vi "Instrument - Manual Object.vi"() -> ()   [LabVIEW 2013, in "Instrument Workspace Objects.lvlib"]
doc: "Sample numeric display item."
uses:
  Instrument Workspace Objects.llb/Instrument Workspace Objects.lvlib
  NationalInstruments.VeriStand.SystemStorage
  Instrument Workspace Objects.llb/Instrument CD Host API.lvlib
panel:
  out "Device":string
  in  "NIVS.System Definition Root":refnum<k24>
  out "Error Report":errorcluster
  in  "Response?":bool
  out "Timed Out?":bool
  out "Response":string
  in  "Send":bool
  in  "Wait Value":dbl=100.0 format="%#_p"
  in  "Wait Type":enum16{"Byte Count", "Wait sec"}(ring)
  in  "Command":string
  in  "Item.Data":T1
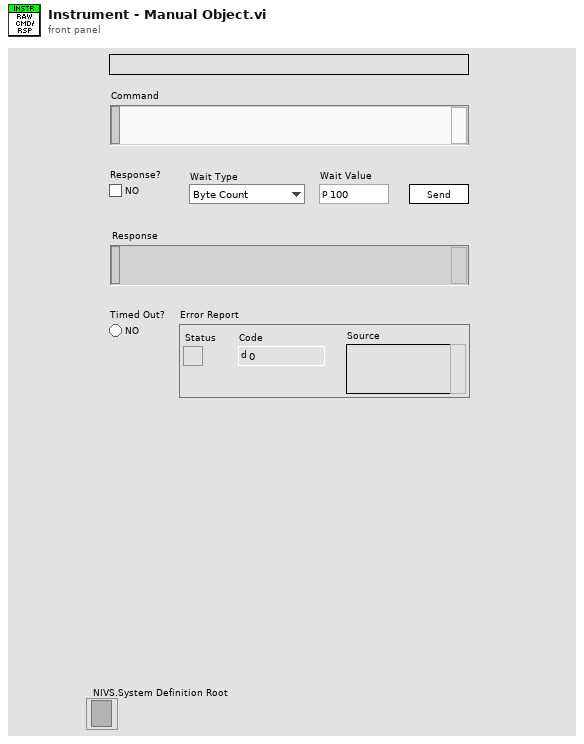
[diagram p1: front panel]
types:
  T1 = cluster{"Template VI":string, "Position X":i32, "Position Y":i32, "Custom":string, "Show Title Bar":bool, "ID":i32, "Always On Top":bool, "Allow Resize":bool, "Allow Minimize":bool, "Allow Close":bool, "Size to Screen":bool, "Screen.ID":i32, "State":enum16{"Normal", "New"}, "Title":string, "Window Bounds":cluster{"[0]":i16, "[1]":i16, "[2]":i16, "[3]":i16}, "Channel Ref":u64, "Unit":string, "Default Units?":bool, "Flash Limit?":bool, "Color 1":u32, "Color 2":u32, "Color 3":u32, "Color 4":u32, "Bck Color":u32, "Fore Color":u32, "Limit 1":dbl, "Limit 2":dbl, "Limit 3":dbl, "Limit 4":dbl, "Limit Mode 1":i32, "Limit Mode 2":i32, "Limit Mode 3":i32, "Limit Mode 4":i32, "Scale Precision":i32, "Scale Min":dbl, "Scale Max":dbl, "Format":i32, "Precision":i32, "Background Type":i32, "IDs":i32[], "Units":string[], "Labels":string[], "Scale Factor":dbl, "Scale Offset":dbl, "YScale Index":u32[], "XScale":cluster{"Format":u8, "Precision":u8, "Fit":u8, "Label":string, "Use Default Label":bool, "Label Visible":bool, "Min":dbl, "Max":dbl}, "YScales":cluster{"Format":u8, "Precision":u8, "Fit":u8, "Label":string, "Use Default Label":bool, "Label Visible":bool, "Min":dbl, "Max":dbl}[], "Plots":cluster{"Bar Style":u8, "Fill To":i16, "Fill/PtColor":u32, "Line Style":u8, "Line Width":u8, "Color":u32, "Interp":u8, "Point Style":u8}[], "Update Period":dbl, "History Length":dbl, "My.Ref":refnum<vi>, "Is Control?":bool, "Channel Paths":string[], "Custom Data":variant}
  T2 = cluster{"Operation":enum16{"SetCustomData", "DeleteItem"}, "Data":variant}
  T3 = cluster{"connection ID":refnum<k5>, "Meta data":string[]}
  T4 = cluster{"Command":string, "Response Expected?":bool, "Wait Type":enum16{"Byte Count", "Wait sec"}, "Wait Value":dbl}
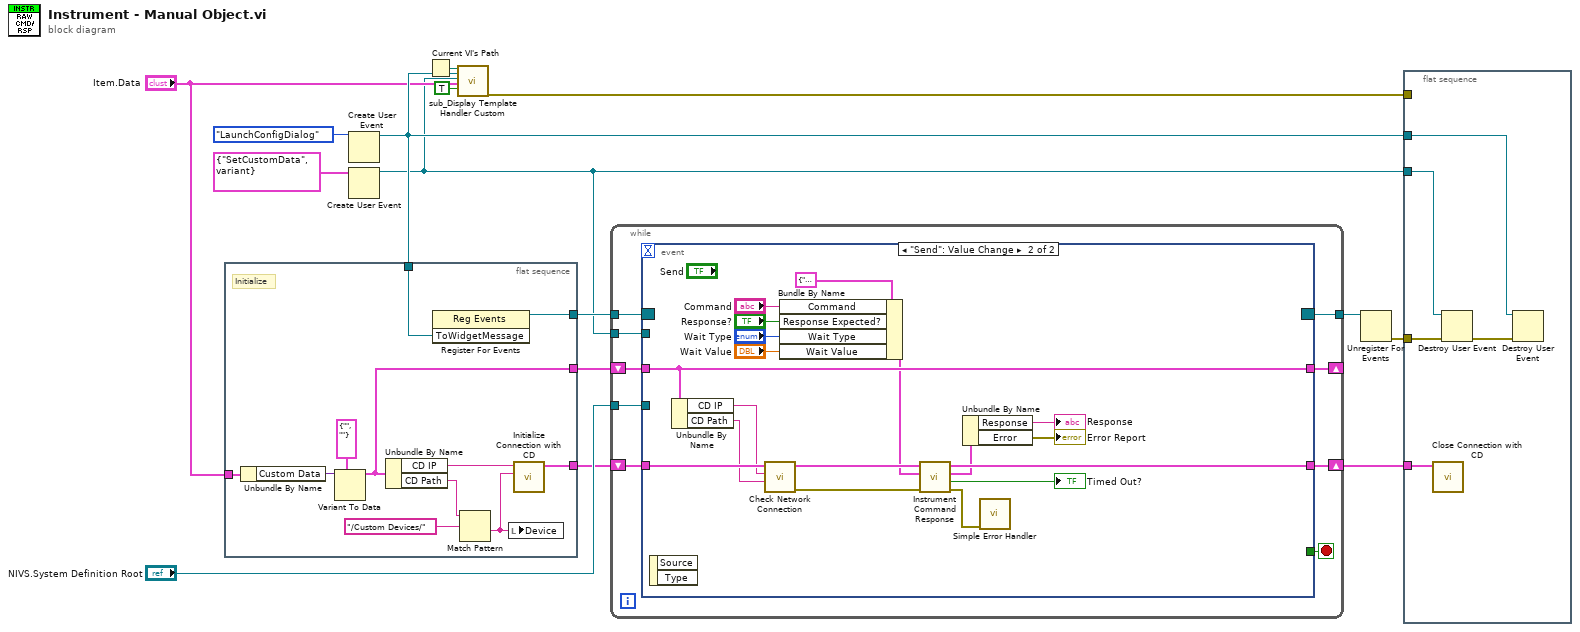
[diagram p0: block diagram]
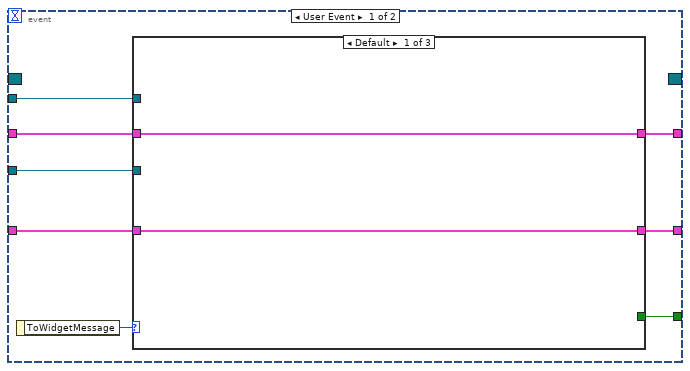
[diagram p2: hidden frame]
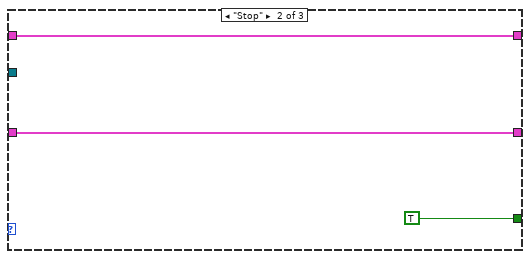
[diagram p3: hidden frame]
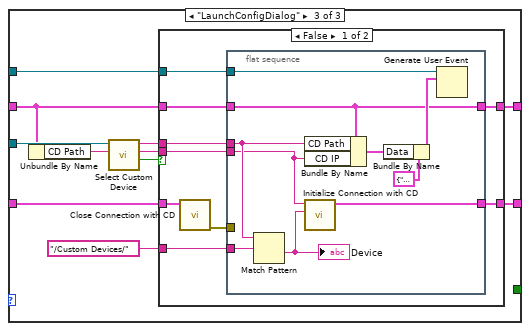
[diagram p4: hidden frame]
diagram:
  n1 = flat-sequence {
    tunnel: [w26] -> w13
    tunnel: w10 -> [w25]
    tunnel: "Item.Data" -> [w24]
    tunnel: [w17] -> w3
    tunnel: [w16] -> w2
    frame #0 {
      # "Initialize"
      n2 = Unbundle By Name(w24) -> ("Custom Data"=w23:variant)
      n3 = Variant To Data(type=cluster{"CD Path":string, "CD IP":string} {"CD Path"="", "CD IP"=""}, Variant=w23) -> (data=w17:cluster{"CD Path":string, "CD IP":string})  [unwired: 1 in, 1 out]
      n4 = Unbundle By Name(w17) -> ("CD IP"=w20:string, "CD Path"=w18:string)
      n5 = register-events(w25) -> (reference out=w26:refnum<event-registration>)  [unwired: 2 in, 1 out]
      n6 = Match Pattern(string=w18, regular expression="/Custom Devices/") -> (after substring=w19:string)  [unwired: 1 in, 3 out]
      n7 = local write "Device"(w19) -> ()
      n8 = call "Initialize Connection with CD.vi"("TCP Service"=w19, "IP Address"=w20) -> ("Connection Info Out"=w16:T3)  [unwired: 8 in, 1 out]
    }
  }
  n9 = Create User Event(user event datatype=enum16{"Stop", "LaunchConfigDialog"}."LaunchConfigDialog" ("ToWidgetMessage")) -> (user event=w10:refnum<user-event>)  [unwired: 1 in, 1 out]
  n10 = Create User Event(user event datatype=T2 {"Operation"=enum."SetCustomData", "Data"=variant} ("Data")) -> (user event=w6:refnum<user-event>)  [unwired: 1 in, 1 out]
  n11 = Current VI's Path() -> (path=w8:path)
  n12 = call "sub_Display Template Handler Custom.vi"("Parent.Path"=w8, "ToWidgetEvent"=w10, "ToWorkspace"=w6, "Item.Data"="Item.Data", "Resizable"=TRUE) -> ("error out"=w15:errorcluster)  [unwired: 14 in]
  n13 = while {
    tunnel: w13 -> [w35]
    tunnel: [w33] -> w12
    tunnel: w6 -> [w32]
    tunnel: "NIVS.System Definition Root" -> [w31]
    shift-right: [w27] -> _
    shift-left: w3 -> [w30]
    shift-right: [w29] -> w1
    shift-left: w2 -> [w28]
    stop <- w34 stop-if-true
    n14 = event shown="[1] \"Send\": Value Change" {
      selector: w35 -> [_ _]
      dyn-events: [_ _] -> w33
      timeout: _ -> [_ _]
      tunnel: [w42 _] -> w34
      tunnel: w32 -> [w41 _]
      tunnel: w31 -> [w40 _]
      tunnel: w30 -> [w39 w92]
      tunnel: [w38 w93] -> w29
      tunnel: w28 -> [w37 w98]
      tunnel: [w36 w92] -> w27
      event User Event {
        n15 = event-data() -> ("ToWidgetMessage"=w43:enum16{"Stop", "LaunchConfigDialog"})  [unwired: 1 out]
        n16 = case shown="Default" w43 {
          tunnel: [_ TRUE _] -> w42
          tunnel: w41 -> [_ _ w59]
          tunnel: w40 -> [_ _ w58]
          tunnel: w39 -> [w44 w46 w52]
          tunnel: [w45 w47 w51] -> w38
          tunnel: w37 -> [w45 w47 w50]
          tunnel: [w44 w46 w49] -> w36
          frame Default {
          }
          frame "Stop" {
          }
          frame "LaunchConfigDialog" {
            n17 = Unbundle By Name(w52) -> ("CD Path"=w57:string)
            n18 = call "Select Custom Device.vi"("CD Path"=w57, "NIVS.System Definition Root"=w58) -> ("Cancelled?"=w56:bool, "IP Address"=w55:string, "Custom Device Path Out"=w54:string)  [unwired: 7 in]
            n19 = case shown="False" w56 {
              tunnel: w59 -> [w68 _]
              tunnel: w55 -> [w64 _]
              tunnel: w54 -> [w66 _]
              tunnel: "/Custom Devices/" ("regular expression") -> [w67 _]
              tunnel: w52 -> [w65 w79]
              tunnel: [w63 w80] -> w51
              tunnel: w50 -> [w62 w80]
              tunnel: [w60 w79] -> w49
              frame False {
                n20 = call "Close Connection with CD.vi"("Connection Info Out"=w62) -> ("error out"=w61:errorcluster)  [unwired: 10 in]
                n21 = flat-sequence {
                  tunnel: w68 -> [w78]
                  tunnel: w67 -> [w75]
                  tunnel: w66 -> [w74]
                  tunnel: w65 -> [w69]
                  tunnel: w64 -> [w72]
                  tunnel: [w70] -> w63
                  tunnel: w61 -> [_]
                  tunnel: [w69] -> w60
                  frame #0 {
                    n22 = Match Pattern(string=w74, regular expression=w75) -> (after substring=w73:string)  [unwired: 1 in, 3 out]
                    "Device" <- w73
                    n23 = Bundle By Name(cluster=w69, "CD Path"=w74, "CD IP"=w72) -> (w71:cluster{"CD Path":string, "CD IP":string})
                    n24 = call "Initialize Connection with CD.vi"("TCP Service"=w73, "IP Address"=w72) -> ("Connection Info Out"=w70:T3)  [unwired: 8 in, 1 out]
                    n25 = Bundle By Name(cluster=T2 {"Operation"=enum."SetCustomData", "Data"=variant} ("event data"), "Data"=w71) -> (w76:T2)
                    n26 = Generate User Event(user event=w78, event data cluster=w76) -> ()  [unwired: 2 in, 2 out]
                  }
                }
              }
              frame True {
              }
            }
          }
        }
      }
      event "Send": Value Change {
        n27 = event-data() -> ()  [unwired: 3 out]
        n28 = Unbundle By Name(w92) -> ("CD IP"=w97:string, "CD Path"=w96:string)
        n29 = call "Check Network Connection.vi"("CD Path"=w96, "IP Address"=w97, "Connection Info"=w98) -> ("error out"=w94:errorcluster, "Connection Info Out"=w95:T3)  [unwired: 7 in]
        n30 = Bundle By Name(cluster=T4 {"Command"="", "Response Expected?"=FALSE, "Wait Type"=enum."Byte Count", "Wait Value"=0.0} ("Command Parameters"), "Command"="Command", "Response Expected?"="Response?", "Wait Type"="Wait Type", "Wait Value"="Wait Value") -> (w87:T4)
        n31 = call "Instrument Command Response.vi"("error in (no error)"=w94, "Command Parameters"=w87, "Connection Info"=w95) -> ("error out"=w82:errorcluster, "Timed Out?"=→"Timed Out?":bool, "Response"=w85:cluster{"Response":string, "Error":errorcluster}, "Connection Info Out"=w93:T3)  [unwired: 5 in]
        n32 = Unbundle By Name(w85) -> ("Response"=→"Response":string, "Error"=→"Error Report":errorcluster)
        n33 = call "Simple Error Handler.vi"("error in (no error)"=w82) -> ()  [unwired: 4 in, 5 out]
      }
    }
  }
  n34 = Unregister For Events(event registration refnum=w12) -> (error out=w11:errorcluster)  [unwired: 1 in]
  n35 = flat-sequence {
    tunnel: w15 -> [_]
    tunnel: w11 -> [w100]
    tunnel: w10 -> [w103]
    tunnel: w6 -> [w102]
    tunnel: w1 -> [w101]
    frame #0 {
      n36 = call "Close Connection with CD.vi"("Connection Info Out"=w101) -> ()  [unwired: 10 in, 1 out]
      n37 = Destroy User Event(user event=w102, error in=w100) -> (error out=w99:errorcluster)
      n38 = Destroy User Event(user event=w103, error in=w99) -> ()  [unwired: 1 out]
    }
  }
